vi "FTDI SPI Close.vi"(8 "error in (no error)":errorcluster, 11 "Handler In":u32) -> (0 "error out":errorcluster)   [LabVIEW 2018]
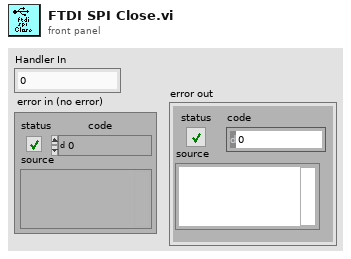
[diagram p1: front panel]
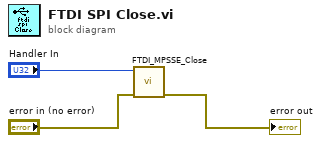
[diagram p0: block diagram]
diagram:
  n1 = call "FTDI_MPSSE_Close.vi"("error in (no error)"="error in (no error)", "Handler"="Handler In") -> ("error out"=→"error out":errorcluster)  [unwired: 9 in]
